vi "ACT_LabVIEW_2p2_Team072.vi"() -> ()   [LabVIEW 2016]
uses:
  <vilib>/express/express arith-compare/Formula/XNode/ExpressFormulaBlockNode.xnode
panel:
  out "Roots Type":string
  in  "c":dbl
  in  "b":dbl
  in  "a":dbl
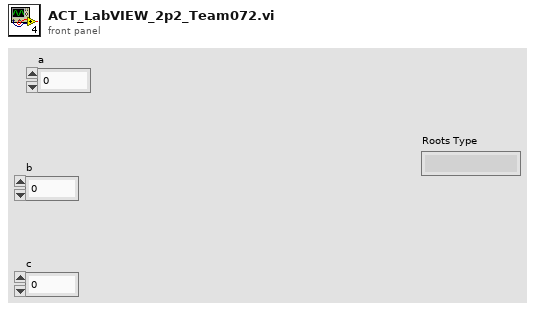
[diagram p1: front panel]
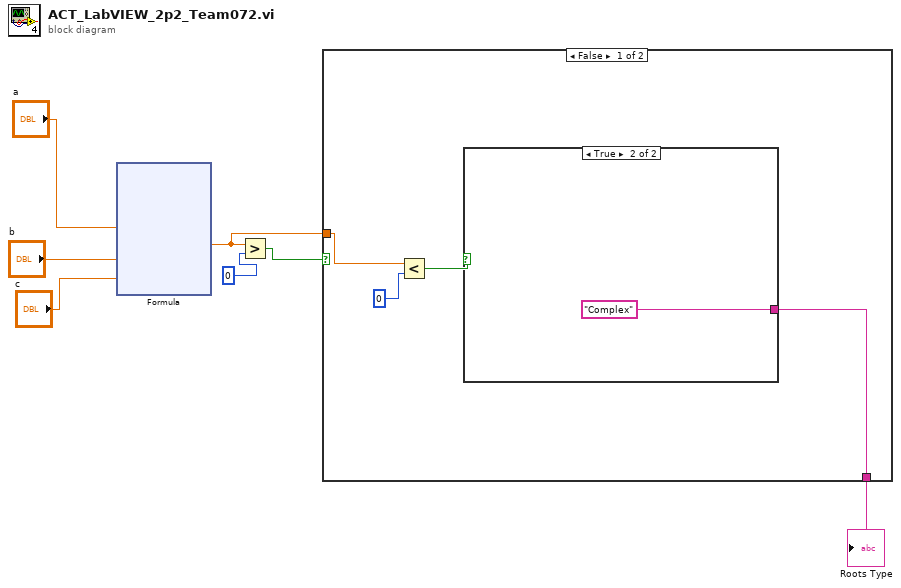
[diagram p0: block diagram]
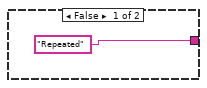
[diagram p2: hidden frame]
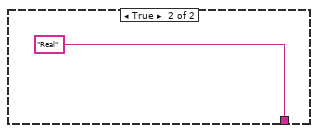
[diagram p3: hidden frame]
diagram:
  n1 = xnode "Formula"("a"="a", "b"="b", "c"="c") -> ("Result"=w1:dbl)  [unwired: 1 in, 1 out]
  n2 = Greater?(x=w1, y=0) -> (0:w3:bool)
  n3 = case shown="False" w3 {
    tunnel: [w8 "Real"] -> w2
    tunnel: w1 -> [w11 _]
    frame False {
      n4 = Less?(x=w11, y=0) -> (x < y?=w9:bool)
      n5 = case shown="True" w9 {
        tunnel: ["Repeated" "Complex"] -> w8
        frame False {
        }
        frame True {
        }
      }
    }
    frame True {
    }
  }
  "Roots Type" <- w2
